vi "Write Scaling.vi"(8 "error in (no error)":errorcluster, 10 "Scaling":dbl, 11 "Configure Scaling Msg in":refnum<class "Configure Scaling Msg.lvclass">) -> (0 "error out":errorcluster, 3 "Configure Scaling Msg out":refnum<class "Configure Scaling Msg.lvclass">)   [LabVIEW 2015, in "CS++Motor.lvlib" / "Configure Scaling Msg.lvclass"]
uses:
  Configure Scaling Msg.lvclass
  Configure Scaling Msg.lvclass/Configure Scaling Msg.ctl
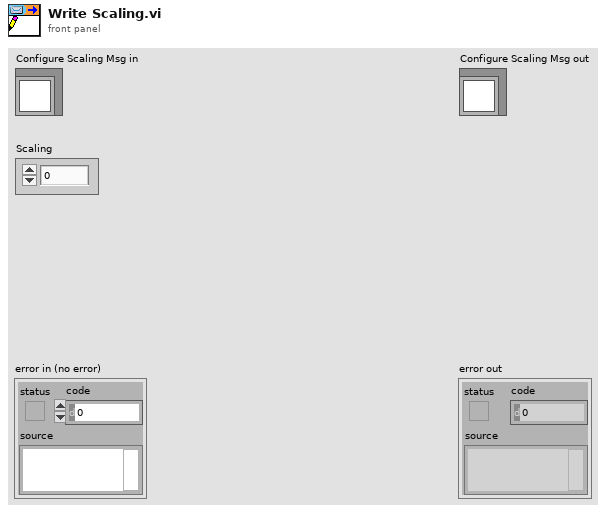
[diagram p1: front panel]
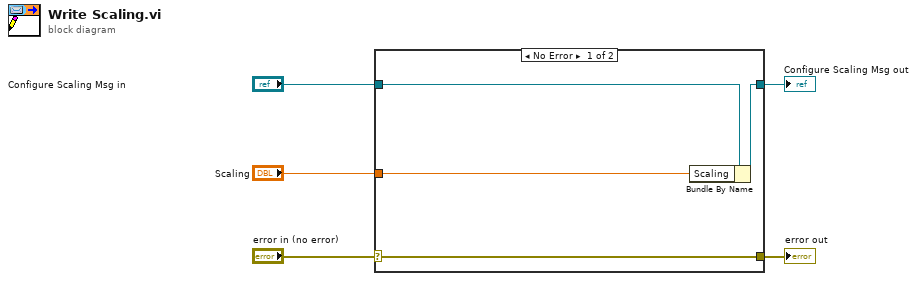
[diagram p0: block diagram]
diagram:
  n1 = case shown="No Error" "error in (no error)" {
    selector: "error in (no error)" -> [w9 w10]
    tunnel: [w9 w10] -> w4
    tunnel: [w7 w11] -> w2
    tunnel: "Configure Scaling Msg in" -> [w8 w11]
    tunnel: "Scaling" -> [w6 _]
    frame No Error {
      n2 = Bundle By Name(cluster=w8, "Scaling"=w6) -> (w7:refnum<class "Configure Scaling Msg.lvclass">)
    }
    frame Error {
    }
  }
  "error out" <- w4
  "Configure Scaling Msg out" <- w2
